vi "Generate DataQ KeyName.vi"(4 "Select":T1, 6 "TaskName":string) -> (7 "DataQ KeyName":string)   [LabVIEW 2017, in "DataQueues.lvclass"]
doc: "Developed by Kevin Thompson\nkevin@thompsonengineering.net\n\nCopyright 2018-2020\nThompson Engineering, LLC"
uses:
  DataQueues.lvclass
  DataTypes/DataQ SelectType--enum.ctl
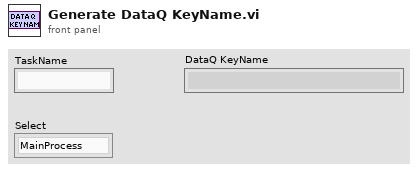
[diagram p1: front panel]
types:
  T1 = typedef "DataQueues.lvclass/DataQ SelectType--enum.ctl" = enum16{"MainProcess", "LogEngine", "LocalDAQThread"}
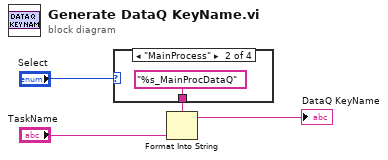
[diagram p0: block diagram]
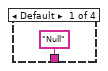
[diagram p2: hidden frame]
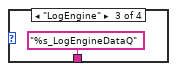
[diagram p3: hidden frame]
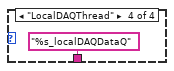
[diagram p4: hidden frame]
diagram:
  n1 = case shown="\"MainProcess\"" "Select" {
    tunnel: ["Null" ("format string") "%s_MainProcDataQ" ("format string") "%s_LogEngineDataQ" ("format string") "%s_localDAQDataQ" ("format string")] -> w1
    frame Default {
    }
    frame "MainProcess" {
    }
    frame "LogEngine" {
    }
    frame "LocalDAQThread" {
    }
  }
  n2 = Format Into String(format string=w1, "TaskName") -> (resulting string=→"DataQ KeyName":string)  [unwired: 2 in, 1 out]
